vi "setDACRS232 V1_2.vi"(3 "error in (no error)":errorcluster, 4 "VISA resource name IN":refnum<visa-resource-name>, 5 "DATA (hexadecimaal)":u16=65535 format="%x", 6 "DAC nr":u8=1) -> (0 "error out":errorcluster, 1 "VISA resource name OUT":refnum<visa-resource-name>)   [LabVIEW 2011]
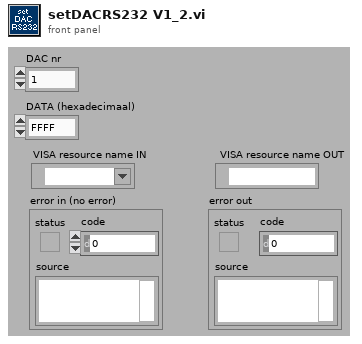
[diagram p1: front panel]
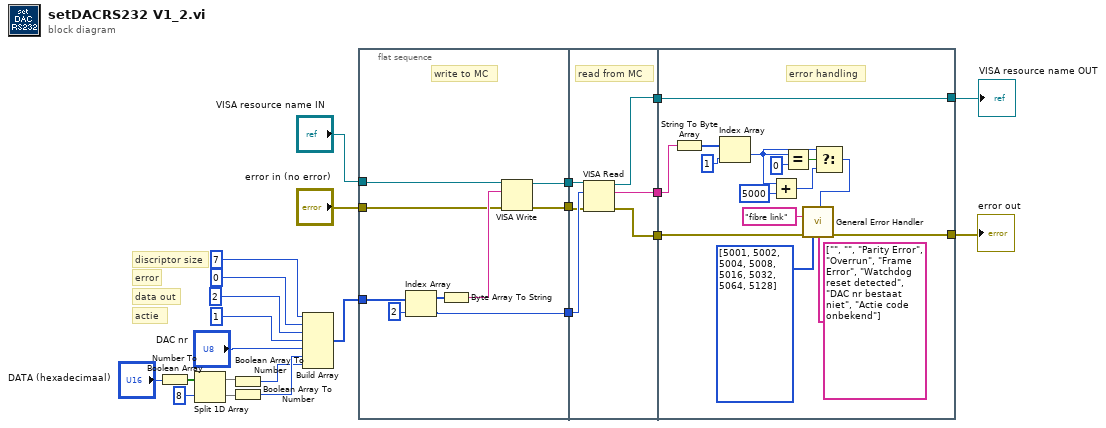
[diagram p0: block diagram]
diagram:
  # "discriptor size"
  # "error"
  # "data out"
  # "actie"
  n1 = Number To Boolean Array(number="DATA (hexadecimaal)") -> (Boolean array=w13:bool[])
  n2 = Split 1D Array(array=w13, index=8) -> (first subarray=w11:bool[], second subarray=w10:bool[])
  n3 = Boolean Array To Number(Boolean array=w11) -> (number=w8:u32)
  n4 = Boolean Array To Number(Boolean array=w10) -> (number=w9:u32)
  n5 = Build Array(u8 7 ("array"), u8 0 ("element"), u8 2 ("element"), u8 1 ("element"), "DAC nr", w9, w8) -> (w7:u32[])
  n6 = flat-sequence {
    tunnel: "VISA resource name IN" -> [w30]
    tunnel: [w28] -> w23
    tunnel: [w25] -> w22
    tunnel: [w26] -> w21
    tunnel: w7 -> [w27]
    tunnel: "error in (no error)" -> [w24]
    tunnel: w23 -> [w37]
    tunnel: w22 -> [w36]
    tunnel: w21 -> [w35]
    tunnel: [w34] -> w20
    tunnel: [w33] -> w2
    tunnel: [w32] -> w1
    tunnel: [w41] -> w3
    tunnel: [w39] -> w4
    tunnel: w20 -> [w41]
    tunnel: w2 -> [w40]
    tunnel: w1 -> [w38]
    frame #0 {
      # "write to MC"
      n7 = Index Array(array=w27, index=2) -> (element=w28:u32)
      n8 = Byte Array To String(unsigned byte array=w27) -> (string=w31:string)
      n9 = VISA Write(VISA resource name=w30, write buffer=w31, error in (no error)=w24) -> (VISA resource name out=w25:refnum<visa-resource-name>, error out=w26:errorcluster)  [unwired: 1 out]
    }
    frame #1 {
      # "read from MC"
      n10 = VISA Read(VISA resource name=w36, byte count=w37, error in (no error)=w35) -> (VISA resource name out=w34:refnum<visa-resource-name>, read buffer=w32:string, error out=w33:errorcluster)  [unwired: 1 out]
    }
    frame #2 {
      # "error handling"
      n11 = String To Byte Array(string=w38) -> (unsigned byte array=w52:u8[])
      n12 = Index Array(array=w52, index=1) -> (element=w43:u8)
      n13 = Add(x=w43, y=u32 5000) -> (x+y=w46:u32)
      n14 = Equal?(x=w43, y=u8 0) -> (x = y?=w44:bool)
      n15 = Select(t=w43, s=w44, f=w46) -> (s? t:f=w45:u32)
      n16 = call <vilib>:"General Error Handler.vi"("[error code] (0)"=w45, "[user-defined codes]"=i32[] [5001, 5002, 5004, 5008, 5016, 5032, 5064, 5128], "[user-defined descriptions]"=string[] ["", "", "Parity Error", "Overrun", "Frame Error", "Watchdog reset detected", "DAC nr bestaat niet", "Actie code onbekend"], "[error source] (\" \")"="fibre link" ("[error source] (\" \")"), "error in (no error)"=w40) -> ("error out"=w39:errorcluster)  [unwired: 6 in, 4 out]
    }
  }
  "error out" <- w4
  "VISA resource name OUT" <- w3
